vi "Message Handler.vi"(11 "Message Handler in":refnum<class "Handler.lvclass">) -> ()   [LabVIEW 2024, in "Ramses Framework.lvlib" / "Handler.lvclass"]
uses:
  Handler.lvclass
  typedefs/Message Format - Cluster.ctl
  Base Server/Server.lvclass
  Service/Service.lvclass
  <vilib>/MediaMongrels Ltd/WebSockets/WebSockets/WebSocket/WebSocket.lvclass
  Ramses Framework.lvlib
panel:
  out "Numeric":i32
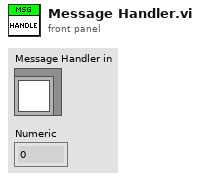
[diagram p1: front panel]
types:
  T1 = typedef "Ramses Framework.lvlib/Handler.lvclass/Message Format - Cluster.ctl" = cluster{"Service":string, "Method":string, "Data":string}
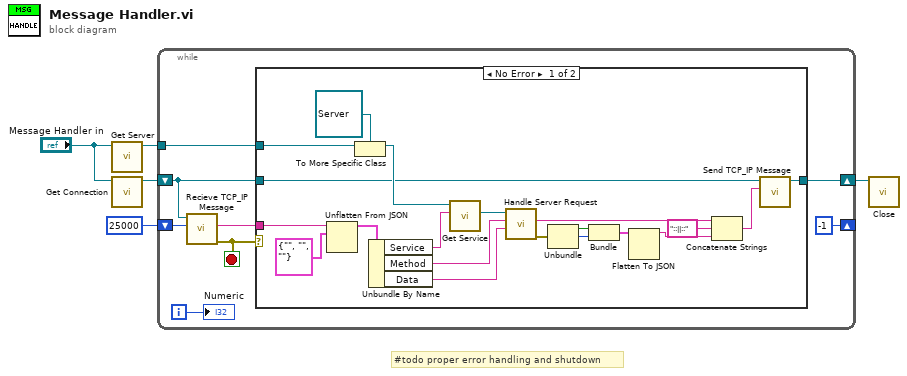
[diagram p0: block diagram]
diagram:
  # "#todo proper error handling and shutdown"
  n1 = call "Get Server.vi"("Handler in"="Message Handler in") -> ("Base Server"=w2:refnum<class "Server.lvclass">)  [unwired: 9 in, 1 out]
  n2 = call "Get Connection.vi"("Handler in"="Message Handler in") -> ("WebSocket"=w3:refnum<class "WebSocket.lvclass">)  [unwired: 9 in, 1 out]
  n3 = while {
    tunnel: w2 -> [w13]
    shift-right: [w10] -> w5
    shift-left: w3 -> [w11]
    shift-right: [-1 ("timeout ms (25000)")] -> _
    shift-left: 25000 ("timeout ms (25000)") -> [w9]
    i -> [w6]
    stop <- w7 stop-if-true
    n4 = call "Recieve TCP_IP Message.vi"("timeout ms (25000)"=w9, "WebSocket in"=w11) -> ("error out"=w7:errorcluster, "Message"=w12:string)  [unwired: 7 in, 1 out]
    n5 = case shown="No Error" w7 {
      tunnel: w13 -> [w33 _]
      tunnel: w12 -> [w25 _]
      tunnel: w11 -> [w17 w34]
      tunnel: [w16 w34] -> w10
      frame No Error {
        n6 = Unflatten From JSON(JSON string=w25, type and defaults=T1 {"Service"="", "Method"="", "Data"=""} ("Cluster")) -> (value=w24:T1)  [unwired: 5 in, 1 out]
        n7 = To More Specific Class(target class=refnum<class "Server.lvclass"> refnum ("Server in"), reference=w33) -> (specific class reference=w19:refnum<class "Server.lvclass">)  [unwired: 1 in, 1 out]
        n8 = Unbundle By Name(w24) -> ("Service"=w15:string, "Method"=w32:string, "Data"=w31:string)
        n9 = call-dynamic "Get Service.vi"("Class Name"=w15, "Server in"=w19) -> ("Service.lvclass"=w27:refnum<class "Service.lvclass">)  [unwired: 7 in, 2 out]
        n10 = call-dynamic "Handle Server Request.vi"("Data"=w31, "Method"=w32, "Service in"=w27) -> ("error out"=w23:errorcluster, "Response"=w30:string)  [unwired: 6 in, 1 out]
        n11 = Unbundle(w23) -> ("status"=w21:bool, "code"=w20:i32)  [unwired: 1 out]
        n12 = Bundle("status"=w21, "code"=w20) -> (w22:cluster{"status":bool, "code":i32})  [unwired: 1 in]
        n13 = Flatten To JSON(anything=w22) -> (JSON string=w29:string)  [unwired: 2 in, 1 out]
        n14 = Concatenate Strings(w30, "::||::" ("Error Seperator"), w29) -> (w28:string)
        n15 = call "Send TCP_IP Message.vi"("Message"=w28, "WebSocket in"=w17) -> ("WebSocket out"=w16:refnum<class "WebSocket.lvclass">)  [unwired: 8 in, 1 out]
      }
      frame Error {
      }
    }
    "Numeric" <- w6
  }
  n16 = call-dynamic "Close.vi"("WebSocket in"=w5) -> ()  [unwired: 10 in, 1 out]
